vi "Target Configuration Options Dialog.vi"(8 "error in":errorcluster, 11 "Target Configuration Options":T1={"NumInBatch"=0, "Target Config Operation"=enum."No Config", "Target Name"="", "Increment Static IPs"=FALSE, "Change Target Name"=FALSE, "Primary NIC"={"MAC address"="", "IP Address Request Mode"=2, "IP address"="", "Subnet mask"="", "Gateway"="", "DNS server"=""}} {"Primary NIC"."IP Address Request Mode" items=["Static"=1, "DHCP/Link-Local"=2, "Link-Local Only"=4, "DHCP Only"=8]}) -> (0 "error out":errorcluster, 1 "Cancelled":bool, 3 "Target Configuration Options":T1={"NumInBatch"=0, "Target Config Operation"=enum."No Config", "Target Name"="", "Increment Static IPs"=FALSE, "Change Target Name"=FALSE, "Primary NIC"={"MAC address"="", "IP Address Request Mode"=2, "IP address"="", "Subnet mask"="", "Gateway"="", "DNS server"=""}} {"Primary NIC"."IP Address Request Mode" items=["Static"=1, "DHCP/Link-Local"=2, "Link-Local Only"=4, "DHCP Only"=8]})   [LabVIEW 2020]
uses:
  Controls/Target Configuration Settings.ctl
  Controls/Target Configuration Operations.ctl
  Controls/Target Network Settings.ctl
  Controls/FP Control Functions.ctl
panel:
  in  "State Variables":cluster{"Target Configuration Options":T1}={"Target Configuration Options"={"NumInBatch"=0, "Target Config Operation"=enum."No Config", "Target Name"="", "Increment Static IPs"=FALSE, "Change Target Name"=FALSE, "Primary NIC"={"MAC address"="", "IP Address Request Mode"=2, "IP address"="", "Subnet mask"="", "Gateway"="", "DNS server"=""}}} {"Target Configuration Options"."Primary NIC"."IP Address Request Mode" items=["Static"=1, "DHCP/Link-Local"=2, "Link-Local Only"=4, "DHCP Only"=8]}
  in  "Change Target Name":bool
  in  "Increment IP":bool
  in  "Deployment Batch Size":u32=1 min=1 max=100
  in  "IP Address Request Mode":i32(ring)=2 items=["Static"=1, "DHCP/Link-Local"=2, "Link-Local Only"=4, "DHCP Only"=8]
  in  "DNS":string
  in  "Gateway":string
  in  "Subnet Mask":string
  in  "IP Address":string
  in  "Target Name (no spaces)":string="RTController"
  in  "Cancel":bool
  in  "OK":bool
  in  "Primary NIC Settings":enum32{"Existing", "Image", "Specify"}(radio)
  # "Batch Image Deployment"
  # "Network Configuration"
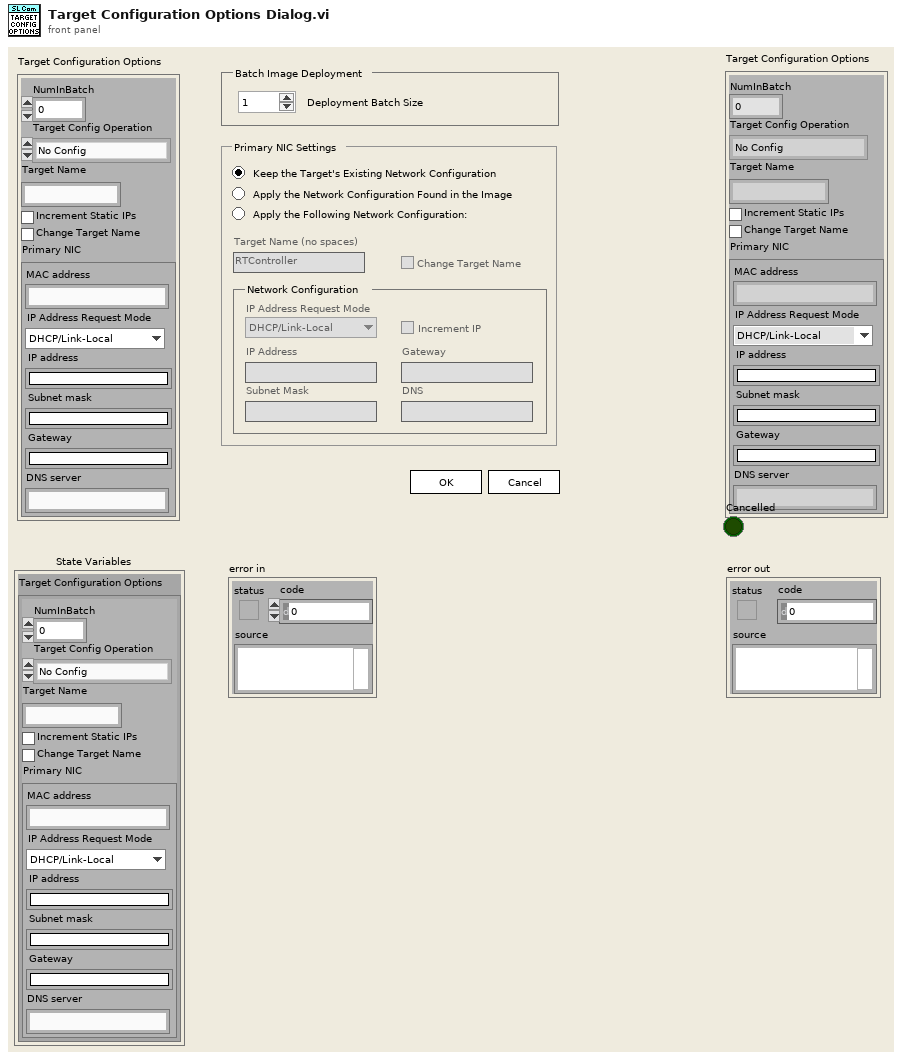
[diagram p1: front panel]
types:
  T1 = typedef "Target Configuration Settings.ctl" = cluster{"NumInBatch":u32, "Target Config Operation":T2, "Target Name":string, "Increment Static IPs":bool, "Change Target Name":bool, "Primary NIC":T3}
  T2 = typedef "Target Configuration Operations.ctl" = enum8{"No Config", "Image Config", "Static Config"}
  T3 = typedef "Target Network Settings.ctl" = cluster{"MAC address":string, "IP Address Request Mode":i32, "IP address":string, "Subnet mask":string, "Gateway":string, "DNS server":string}
  T4 = typedef "FP Control Functions.ctl" = enum16{"Open", "Close", "Bring To Front", "Center"}
  T5 = enum8{"Enabled", "Disabled", "Disabled and Grayed Out"}
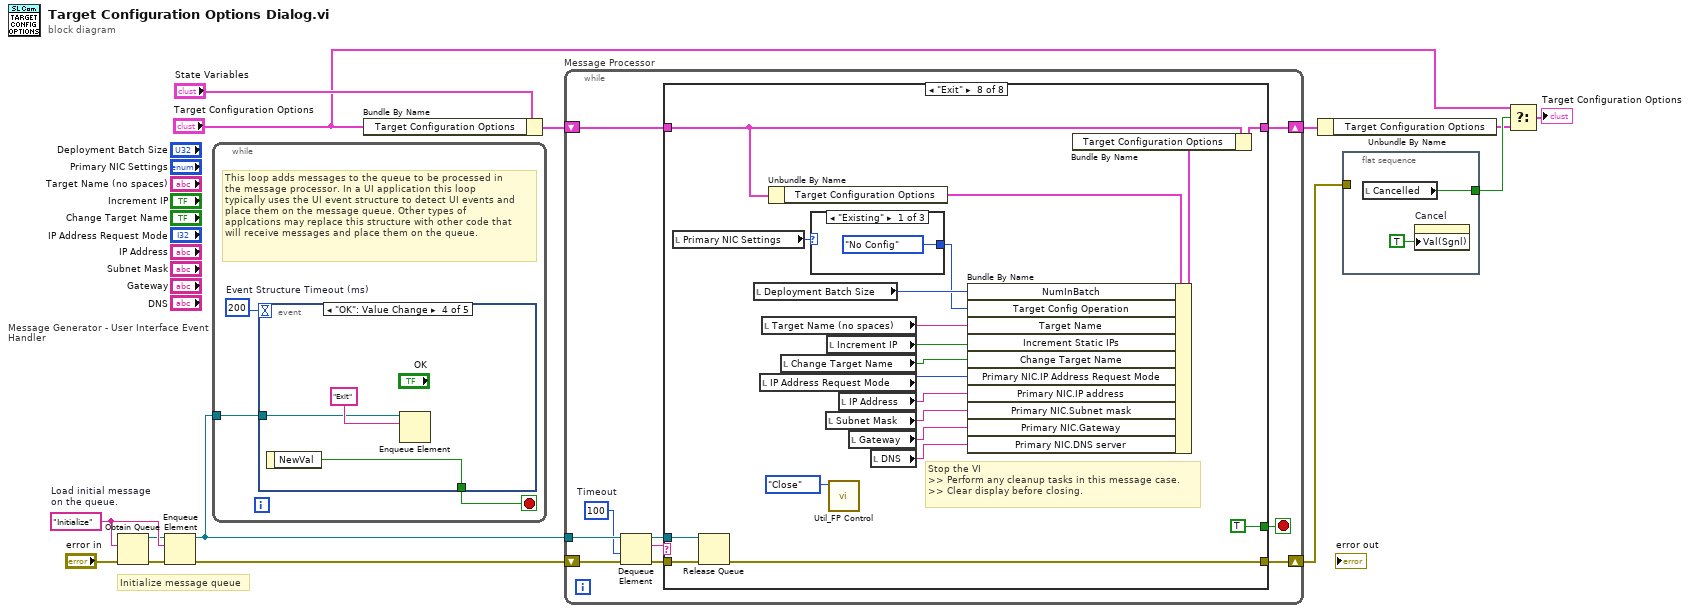
[diagram p0: block diagram]
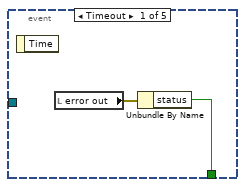
[diagram p2: hidden frame]
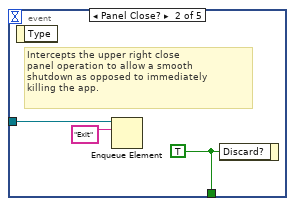
[diagram p3: hidden frame]
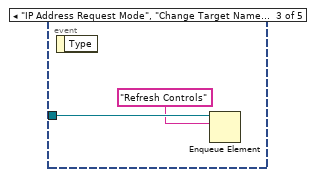
[diagram p4: hidden frame]
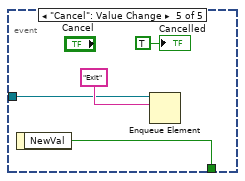
[diagram p5: hidden frame]
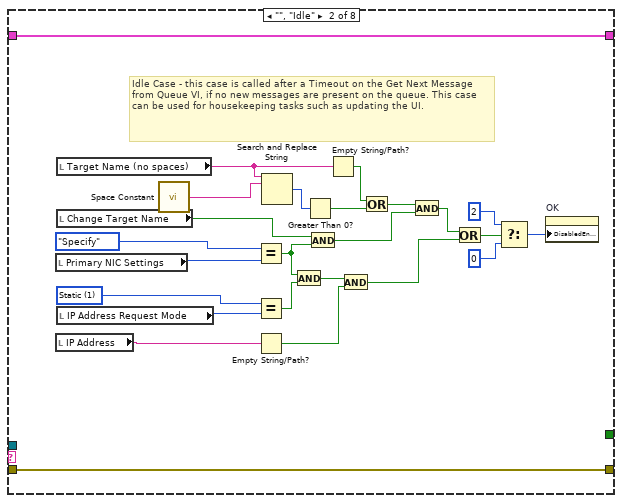
[diagram p7: hidden frame]
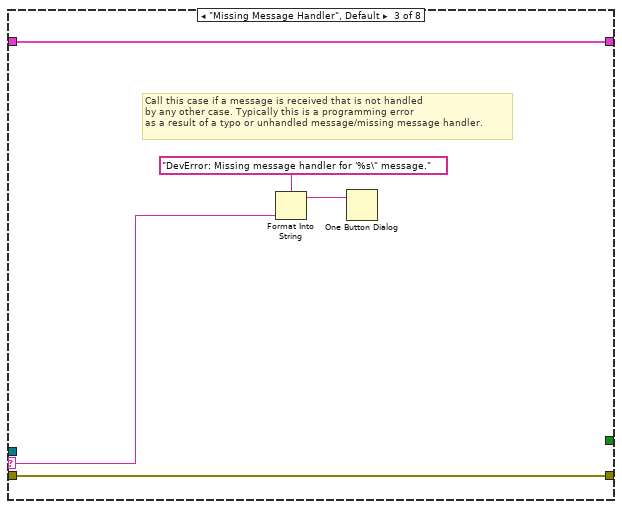
[diagram p8: hidden frame]
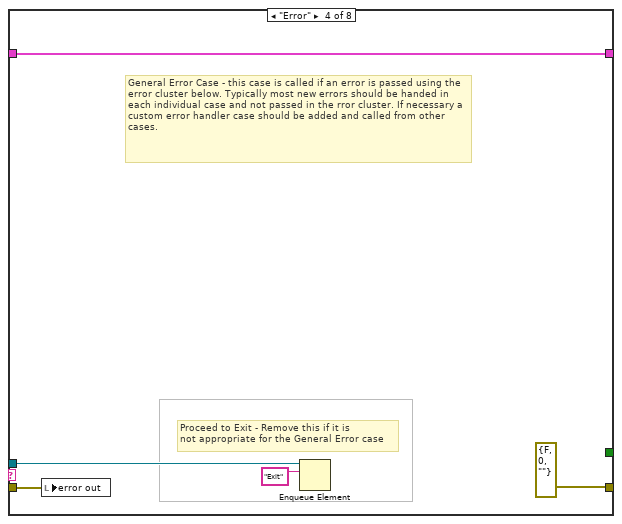
[diagram p9: hidden frame]
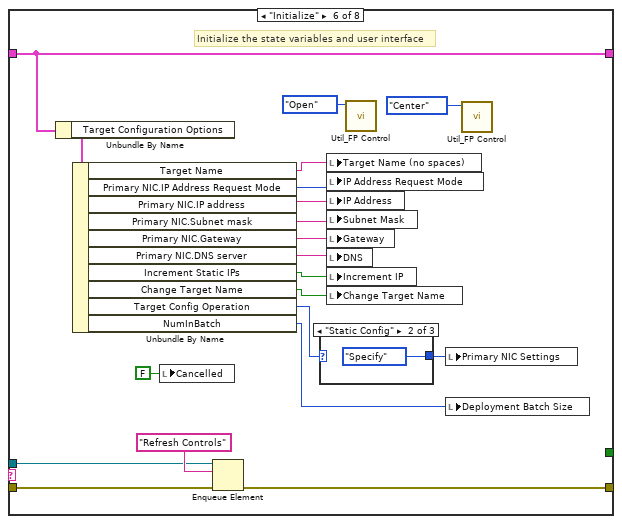
[diagram p11: hidden frame]
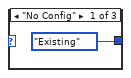
[diagram p12: hidden frame]
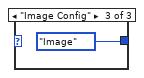
[diagram p13: hidden frame]
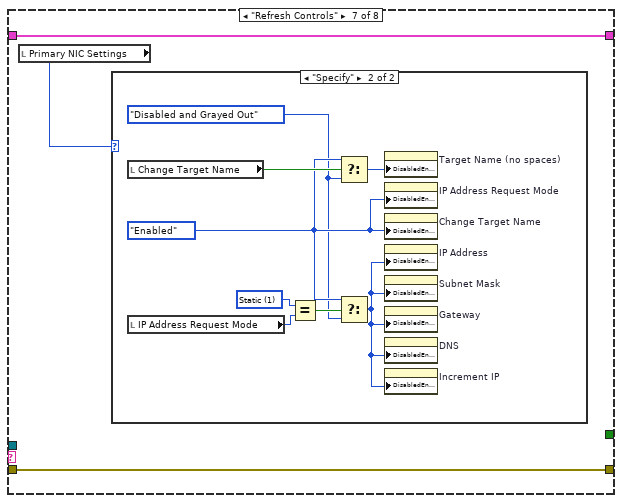
[diagram p14: hidden frame]
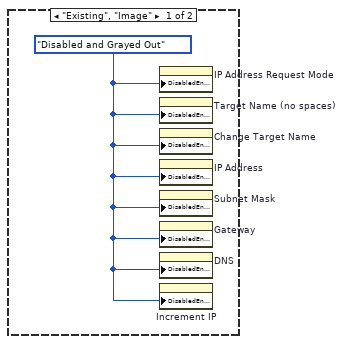
[diagram p15: hidden frame]
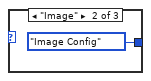
[diagram p16: hidden frame]
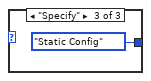
[diagram p17: hidden frame]
diagram:
  w3 = "Initialize"  # Load initial message on the queue.
  # "Initialize message queue"
  n1 = Obtain Queue(element data type=w3, error in (no error)="error in") -> (queue out=w1:refnum<queue>, error out=w14:errorcluster)  [unwired: 3 in, 1 out]
  n2 = Enqueue Element(queue=w1, element=w3, error in (no error)=w14) -> (queue out=w2:refnum<queue>, error out=w4:errorcluster)  [unwired: 1 in, 1 out]
  n3 = while "Message Generator - User Interface Event Handler" {
    tunnel: w2 -> [w15]
    stop <- w16 stop-if-true
    w17 = 200  # Event Structure Timeout (ms)
    # "This loop adds messages to the queue to be processed in\nthe message processor. In a UI application this loop\ntypically uses the UI event structure to detect UI events and\nplace them on the message queue. Other types of\napplcations may replace this structure with other code that\nwill receive messages and place them on the queue."
    n4 = event shown="[3] \"OK\": Value Change" {
      selector: _ -> [_ _ _ _ _]
      dyn-events: _ -> [_ _ _ _ _]
      timeout: w17 -> [_ _ _ _ _]
      tunnel: [w18 w22 _ w25 w29] -> w16
      tunnel: w15 -> [_ w20 w24 w26 w30]
      event Timeout {
        n5 = event-data() -> ()  [unwired: 2 out]
        n6 = local read "error out"() -> (w19:errorcluster)
        n7 = Unbundle By Name(w19) -> ("status"=w18:bool)
      }
      event Panel Close? {
        w22 = TRUE ("Discard?")
        # "Intercepts the upper right close\npanel operation to allow a smooth\nshutdown as opposed to immediately\nkilling the app."
        n8 = event-data() -> ()  [unwired: 2 out]
        n9 = Enqueue Element(queue=w20, element="Exit") -> ()  [unwired: 2 in, 3 out]
        n10 = event-data("Discard?"=w22) -> ()  [unwired: 1 in, 1 out]
      }
      event "IP Address Request Mode", "Change Target Name", "Primary NIC Settings": Value Change {
        n11 = event-data() -> ()  [unwired: 2 out]
        n12 = Enqueue Element(queue=w24, element="Refresh Controls") -> ()  [unwired: 2 in, 3 out]
      }
      event "OK": Value Change {
        n13 = event-data() -> ("NewVal"=w25:bool)  [unwired: 1 out]
        n14 = Enqueue Element(queue=w26, element="Exit") -> ()  [unwired: 2 in, 3 out]
      }
      event "Cancel": Value Change {
        n15 = event-data() -> ("NewVal"=w29:bool)  [unwired: 1 out]
        n16 = Enqueue Element(queue=w30, element="Exit") -> ()  [unwired: 2 in, 3 out]
        "Cancelled" <- TRUE ("Cancelled")
      }
    }
  }
  n17 = Bundle By Name(cluster="State Variables", "Target Configuration Options"="Target Configuration Options") -> (w12:cluster{"Target Configuration Options":T1})
  n18 = while "Message Processor" {
    shift-left: w4 -> [w37]
    shift-right: [w39] -> w9
    tunnel: w2 -> [w33]
    shift-left: w12 -> [w41]
    shift-right: [w40] -> w10
    stop <- w34 stop-if-true
    w32 = 100  # Timeout
    n19 = Dequeue Element(queue=w33, timeout in ms (-1)=w32, error in (no error)=w37) -> (queue out=w38:refnum<queue>, element=w35:string, error out=w36:errorcluster)  [unwired: 1 out]
    n20 = case shown="\"Exit\"" w35 {
      selector: w35 -> [_ _ w71 _ _ _ _ _]
      tunnel: [w43 w68 w73 w78 w80 w92 w106 w118] -> w40
      tunnel: w41 -> [w43 w68 w73 w78 w80 w92 w106 w119]
      tunnel: w38 -> [_ _ _ w76 _ w89 _ w134]
      tunnel: w36 -> [w42 w67 w72 w74 w79 w88 w105 w135]
      tunnel: [w42 w67 w72 errorcluster {"status"=FALSE, "code"=0, "source"=""} ("error out") w79 w87 w105 w133] -> w39
      tunnel: [_ _ _ _ _ _ _ TRUE] -> w34
      frame "---------- Framework Operations ----------" {
        # "Dummy case to add a seperator in the Case Structure menu"
      }
      frame "", "Idle" {
        w45 = 1 items=["Static"=1, "DHCP/Link-Local"=2, "Link-Local Only"=4, "DHCP Only"=8] ("IP Address Request Mode")
        # "Idle Case - this case is called after a Timeout on the Get Next Message from Queue VI, if no new messages are present on the queue. This case can be used for housekeeping tasks such as updating the UI."
        n21 = local read "Primary NIC Settings"() -> (w54:enum32{"Existing", "Image", "Specify"})
        n22 = local read "IP Address"() -> (w64:string)
        n23 = local read "Target Name (no spaces)"() -> (w53:string)
        n24 = local read "Change Target Name"() -> (w49:bool)
        n25 = local read "IP Address Request Mode"() -> (w46:i32)
        n26 = call <vilib>:"Space Constant.vi"() -> ("String"=w66:string)
        n27 = Equal?(x=enum32{"Existing", "Image", "Specify"}."Specify" ("NIC Source"), y=w54) -> (x = y?=w48:bool)
        n28 = Equal?(x=w45, y=w46) -> (x = y?=w44:bool)
        n29 = Empty String/Path?(string/path=w64) -> (empty?=w63:bool)
        n30 = Search and Replace String(input string=w53, search string=w66) -> (number of replacements=w65:i32)  [unwired: 6 in, 3 out]
        n31 = And(x=w48, y=w44) -> (x .and. y?=w62:bool)
        n32 = Greater Than 0?(x=w65) -> (x > 0?=w51:bool)
        n33 = And(x=w49, y=w48) -> (x .and. y?=w47:bool)
        n34 = Empty String/Path?(string/path=w53) -> (empty?=w52:bool)
        n35 = And(x=w62, y=w63) -> (x .and. y?=w60:bool)
        n36 = Or(x=w52, y=w51) -> (x .or. y?=w50:bool)
        n37 = And(x=w50, y=w47) -> (x .and. y?=w61:bool)
        n38 = Or(x=w61, y=w60) -> (x .or. y?=w59:bool)
        n39 = Select(t=2, s=w59, f=0) -> (s? t:f=w56:i32)
        n40 = property on="OK" class="Bool"("DisabledEnum"=w56) -> ()  [unwired: 2 in, 2 out]
      }
      frame "Missing Message Handler", Default {
        # "Call this case if a message is received that is not handled \nby any other case. Typically this is a programming error\nas a result of a typo or unhandled message/missing message handler."
        n41 = Format Into String(format string="DevError: Missing message handler for '%s\" message." ("message"), w71) -> (resulting string=w69:string)  [unwired: 2 in, 1 out]
        n42 = One Button Dialog(message=w69) -> ()  [unwired: 2 out]
      }
      frame "Error" {
        # "Proceed to Exit - Remove this if it is\nnot appropriate for the General Error case"
        # "General Error Case - this case is called if an error is passed using the error cluster below. Typically most new errors should be handed in each individual case and not passed in the rror cluster. If necessary a custom error handler case should be added and called from other cases."
        n43 = local write "error out"(w74) -> ()
        n44 = Enqueue Element(queue=w76, element="Exit") -> ()  [unwired: 2 in, 3 out]
      }
      frame "---------- Generic Operations ----------" {
        # "Dummy case to add a seperator in the Case Structure menu"
      }
      frame "Initialize" {
        # "Initialize the state variables and user interface"
        n45 = Unbundle By Name(w92) -> ("Target Configuration Options"=w91:T1)
        n46 = Unbundle By Name(w91) -> ("Target Name"=w99:string, "Primary NIC.IP Address Request Mode"=w100:i32, "Primary NIC.IP address"=w98:string, "Primary NIC.Subnet mask"=w97:string, "Primary NIC.Gateway"=w96:string, "Primary NIC.DNS server"=w95:string, "Increment Static IPs"=w94:bool, "Change Target Name"=w93:bool, "Target Config Operation"=w86:T2, "NumInBatch"=w82:u32)
        n47 = local write "Cancelled"(FALSE ("Cancelled")) -> ()
        n48 = Enqueue Element(queue=w89, element="Refresh Controls", error in (no error)=w88) -> (error out=w87:errorcluster)  [unwired: 1 in, 2 out]
        n49 = case shown="\"Static Config\"" w86 {
          tunnel: [enum32{"Existing", "Image", "Specify"}."Existing" ("NIC Source") enum32{"Existing", "Image", "Specify"}."Specify" ("NIC Source") enum32{"Existing", "Image", "Specify"}."Image" ("NIC Source")] -> w81
          frame "No Config" {
          }
          frame "Static Config" {
          }
          frame "Image Config" {
          }
        }
        n50 = local write "Target Name (no spaces)"(w99) -> ()
        n51 = local write "IP Address Request Mode"(w100) -> ()
        n52 = local write "IP Address"(w98) -> ()
        n53 = local write "Subnet Mask"(w97) -> ()
        n54 = local write "Gateway"(w96) -> ()
        n55 = local write "DNS"(w95) -> ()
        n56 = local write "Increment IP"(w94) -> ()
        n57 = local write "Change Target Name"(w93) -> ()
        n58 = call "Util_FP Control.vi"("Function"=FP_Control_Functions."Open") -> ()  [unwired: 10 in, 1 out]
        n59 = local write "Primary NIC Settings"(w81) -> ()
        n60 = local write "Deployment Batch Size"(w82) -> ()
        n61 = call "Util_FP Control.vi"("Function"=FP_Control_Functions."Center") -> ()  [unwired: 10 in, 1 out]
      }
      frame "Refresh Controls" {
        n62 = local read "Primary NIC Settings"() -> (w104:enum32{"Existing", "Image", "Specify"})
        n63 = case shown="\"Specify\"" w104 {
          frame "Existing", "Image" {
            w107 = T5."Disabled and Grayed Out" ("Disabled")
            n64 = property on="IP Address Request Mode" class="Ring (strict)"("DisabledEnum"=w107) -> ()  [unwired: 2 in, 2 out]
            n65 = property on="Target Name (no spaces)" class="Str"("DisabledEnum"=w107) -> ()  [unwired: 2 in, 2 out]
            n66 = property on="Change Target Name" class="Bool (strict)"("DisabledEnum"=w107) -> ()  [unwired: 2 in, 2 out]
            n67 = property on="IP Address" class="Str"("DisabledEnum"=w107) -> ()  [unwired: 2 in, 2 out]
            n68 = property on="Subnet Mask" class="Str"("DisabledEnum"=w107) -> ()  [unwired: 2 in, 2 out]
            n69 = property on="Gateway" class="Str"("DisabledEnum"=w107) -> ()  [unwired: 2 in, 2 out]
            n70 = property on="DNS" class="Str"("DisabledEnum"=w107) -> ()  [unwired: 2 in, 2 out]
            n71 = property on="Increment IP" class="Bool (strict)"("DisabledEnum"=w107) -> ()  [unwired: 2 in, 2 out]
          }
          frame "Specify" {
            w112 = 1 items=["Static"=1, "DHCP/Link-Local"=2, "Link-Local Only"=4, "DHCP Only"=8] ("IP Address Request Mode")
            w108 = T5."Disabled and Grayed Out" ("Disabled")
            w109 = T5."Enabled" ("Disabled")
            n72 = local read "Change Target Name"() -> (w114:bool)
            n73 = local read "IP Address Request Mode"() -> (w111:i32)
            n74 = Equal?(x=w112, y=w111) -> (x = y?=w110:bool)
            n75 = Select(t=w109, s=w114, f=w108) -> (s? t:f=w113:T5)
            n76 = Select(t=w109, s=w110, f=w108) -> (s? t:f=w115:T5)
            n77 = property on="Target Name (no spaces)" class="Str"("DisabledEnum"=w113) -> ()  [unwired: 2 in, 2 out]
            n78 = property on="IP Address Request Mode" class="Ring (strict)"("DisabledEnum"=w109) -> ()  [unwired: 2 in, 2 out]
            n79 = property on="Change Target Name" class="Bool (strict)"("DisabledEnum"=w109) -> ()  [unwired: 2 in, 2 out]
            n80 = property on="IP Address" class="Str"("DisabledEnum"=w115) -> ()  [unwired: 2 in, 2 out]
            n81 = property on="Subnet Mask" class="Str"("DisabledEnum"=w115) -> ()  [unwired: 2 in, 2 out]
            n82 = property on="Gateway" class="Str"("DisabledEnum"=w115) -> ()  [unwired: 2 in, 2 out]
            n83 = property on="DNS" class="Str"("DisabledEnum"=w115) -> ()  [unwired: 2 in, 2 out]
            n84 = property on="Increment IP" class="Bool (strict)"("DisabledEnum"=w115) -> ()  [unwired: 2 in, 2 out]
          }
        }
      }
      frame "Exit" {
        # "Stop the VI\n>> Perform any cleanup tasks in this message case.\n>> Clear display before closing."
        n85 = local read "Primary NIC Settings"() -> (w121:enum32{"Existing", "Image", "Specify"})
        n86 = Release Queue(queue=w134, error in (no error)=w135) -> (error out=w133:errorcluster)  [unwired: 1 in, 2 out]
        n87 = local read "Deployment Batch Size"() -> (w123:u32)
        n88 = local read "IP Address Request Mode"() -> (w127:i32)
        n89 = local read "Target Name (no spaces)"() -> (w124:string)
        n90 = Unbundle By Name(w119) -> ("Target Configuration Options"=w120:T1)
        n91 = local read "Change Target Name"() -> (w126:bool)
        n92 = case shown="\"Existing\"" w121 {
          tunnel: [Target_Configuration_Operations."No Config" ("Target Config Operation") Target_Configuration_Operations."Image Config" ("Target Config Operation") Target_Configuration_Operations."Static Config" ("Target Config Operation")] -> w122
          frame "Existing" {
          }
          frame "Image" {
          }
          frame "Specify" {
          }
        }
        n93 = local read "Subnet Mask"() -> (w129:string)
        n94 = local read "Increment IP"() -> (w125:bool)
        n95 = call "Util_FP Control.vi"("Function"=FP_Control_Functions."Close") -> ()  [unwired: 10 in, 1 out]
        n96 = local read "IP Address"() -> (w128:string)
        n97 = local read "Gateway"() -> (w130:string)
        n98 = local read "DNS"() -> (w131:string)
        n99 = Bundle By Name(cluster=w120, "NumInBatch"=w123, "Target Config Operation"=w122, "Target Name"=w124, "Increment Static IPs"=w125, "Change Target Name"=w126, "Primary NIC.IP Address Request Mode"=w127, "Primary NIC.IP address"=w128, "Primary NIC.Subnet mask"=w129, "Primary NIC.Gateway"=w130, "Primary NIC.DNS server"=w131) -> (w117:T1)
        n100 = Bundle By Name(cluster=w119, "Target Configuration Options"=w117) -> (w118:cluster{"Target Configuration Options":T1})
      }
    }
  }
  n101 = Unbundle By Name(w10) -> ("Target Configuration Options"=w7:T1)
  n102 = flat-sequence {
    tunnel: w9 -> [_]
    tunnel: [w140] -> w8
    frame #0 {
      n103 = local read "Cancelled"() -> (w140:bool)
      n104 = property on="Cancel" class="Bool"("Val(Sgnl)"=TRUE) -> ()  [unwired: 2 in, 2 out]
    }
  }
  n105 = Select(t="Target Configuration Options", s=w8, f=w7) -> (s? t:f=→"Target Configuration Options":T1)
